vi "Find Ref by Name (SubVI).vi"(0 "Control Refs":cluster{"Label Name":string, "Ref":refnum<vi>}[](array[cluster]), 2 "Label Name":string, 11 "Error IN":errorcluster) -> (4 "Control Reference":refnum<vi>, 15 "Error OUT":errorcluster)   [LabVIEW 2012]
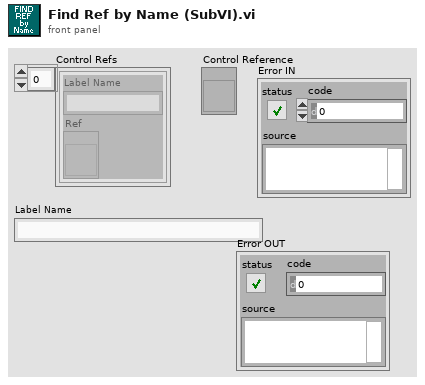
[diagram p1: front panel]
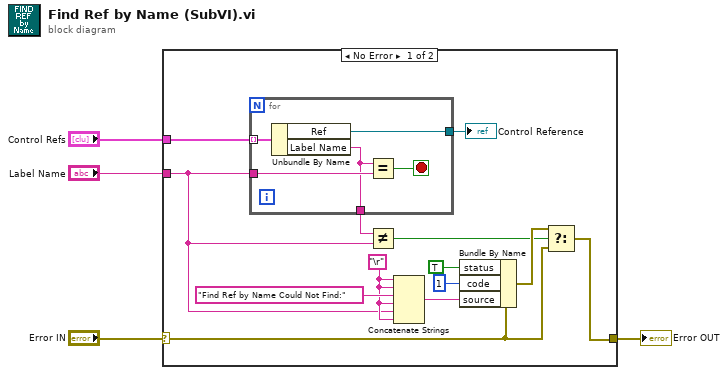
[diagram p0: block diagram]
diagram:
  n1 = case shown="No Error" "Error IN" {
    selector: "Error IN" -> [w13 w23]
    tunnel: "Control Refs" -> [w17 _]
    tunnel: "Label Name" -> [w5 _]
    tunnel: [w14 w23] -> w1
    frame No Error {
      w6 = "\r"
      n2 = for {
        tunnel: w17 -> [w22] mode=indexing
        tunnel: w5 -> [w21]
        tunnel: [w20] -> w16
        tunnel: [w18] -> w15
        stop <- w19 stop-if-true
        n3 = Unbundle By Name(w22) -> ("Ref"=w20:refnum<vi>, "Label Name"=w18:string)
        n4 = Equal?(x=w18, y=w21) -> (x = y?=w19:bool)
      }
      "Control Reference" <- w16
      n5 = Not Equal?(x=w15, y=w5) -> (x != y?=w8:bool)
      n6 = Concatenate Strings(w6, w6, "Find Ref by Name Could Not Find:", w6, w5, w6) -> (w10:string)
      n7 = Bundle By Name(cluster=w13, "status"=TRUE, "code"=1, "source"=w10) -> (w9:errorcluster)
      n8 = Select(t=w9, s=w8, f=w13) -> (s? t:f=w14:errorcluster)
    }
    frame Error {
    }
  }
  "Error OUT" <- w1
